vi "_readBoolSpecItem.vi"(7 "Error If Not Found":bool, 8 "error in (no error)":errorcluster, 9 "Default Value":bool, 10 "Name":string, 11 "Build Spec In":refnum<class "tBSONDocument.lvclass">) -> (0 "error out":errorcluster, 1 "Value":bool, 2 "Found":bool, 3 "Build Spec Out":refnum<class "tBSONDocument.lvclass">)   [LabVIEW 2013, in "LVAutomationListener.lvlib" / "LVAutomationListener.lvclass"]
uses:
  LVAutomationListener.lvclass
  BSON/tBSONDocument/tBSONDocument.lvclass
  _status.ctl
  BSON/tBSONDocument/getBooleanValue.vi
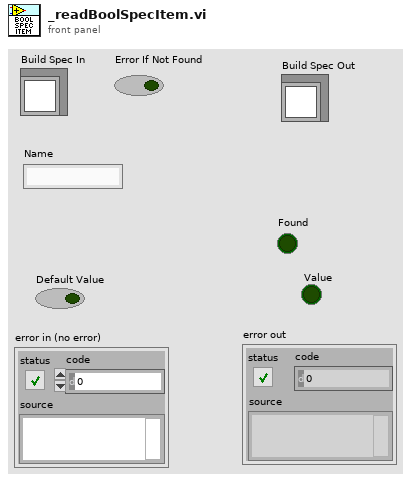
[diagram p1: front panel]
types:
  T1 = typedef "LVAutomationListener.lvlib/LVAutomationListener.lvclass/_status.ctl" = enum16{"Missing Argument", "Unknown Command", "Missing Build Spec Item", "Bad Type", "Compiler Aborted"}
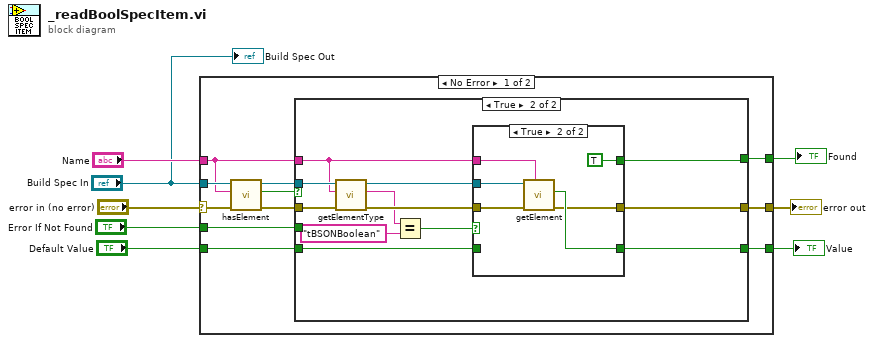
[diagram p0: block diagram]
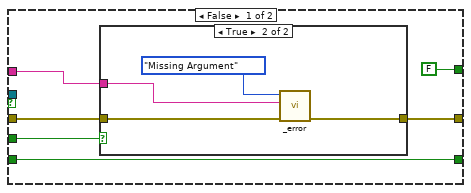
[diagram p2: hidden frame]
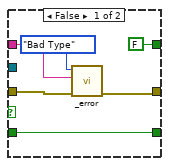
[diagram p4: hidden frame]
diagram:
  n1 = case shown="No Error" "error in (no error)" {
    selector: "error in (no error)" -> [w19 w56]
    tunnel: "Build Spec In" -> [w18 _]
    tunnel: "Name" -> [w13 _]
    tunnel: "Default Value" -> [w14 w55]
    tunnel: [w12 w55] -> w5
    tunnel: [w11 w56] -> w4
    tunnel: "Error If Not Found" -> [w10 _]
    tunnel: [w9 _] -> w1
    frame No Error {
      n2 = call "hasElement.vi"("error in (no error)"=w19, "Name"=w13, "tBSONDocument in"=w18) -> ("error out"=w16:errorcluster, "hasElement"=w17:bool, "tBSONDocument out"=w15:refnum<class "tBSONDocument.lvclass">)  [unwired: 6 in]
      n3 = case shown="True" w17 {
        tunnel: w16 -> [w23 w39]
        tunnel: w15 -> [_ w40]
        tunnel: w14 -> [w25 w34]
        tunnel: w13 -> [w22 w38]
        tunnel: [w25 w42] -> w12
        tunnel: [w21 w41] -> w11
        tunnel: w10 -> [w24 _]
        tunnel: [FALSE w33] -> w9
        frame False {
          n4 = case shown="True" w24 {
            tunnel: w23 -> [w26 w30]
            tunnel: w22 -> [_ w28]
            tunnel: [w26 w27] -> w21
            frame False {
            }
            frame True {
              n5 = call "_error.vi"("error in (no error)"=w30, "Additional message"=w28, "Status"=_status."Missing Argument") -> ("error out"=w27:errorcluster)  [unwired: 8 in]
            }
          }
        }
        frame True {
          n6 = call "getElementType.vi"("error in (no error)"=w39, "Name"=w38, "tBSONDocument in"=w40) -> ("error out"=w37:errorcluster, "TypeClass"=w31:string, "tBSONDocument out"=w36:refnum<class "tBSONDocument.lvclass">)  [unwired: 6 in]
          n7 = Equal?(x=w31, y="tBSONBoolean" ("x")) -> (x = y?=w35:bool)
          n8 = case shown="True" w35 {
            tunnel: [w44 w54] -> w42
            tunnel: [w45 w53] -> w41
            tunnel: w38 -> [w47 w52]
            tunnel: w37 -> [w48 w51]
            tunnel: w36 -> [_ w50]
            tunnel: w34 -> [w44 _]
            tunnel: [FALSE TRUE] -> w33
            frame False {
              n9 = call "_error.vi"("error in (no error)"=w48, "Additional message"=w47, "Status"=_status."Bad Type") -> ("error out"=w45:errorcluster)  [unwired: 8 in]
            }
            frame True {
              n10 = call-poly "getElement.vi"("Name"=w52, "error in (no error)"=w51, "tBSONDocument in"=w50) -> ("error out"=w53:errorcluster, "Value"=w54:bool)  [unwired: 6 in, 1 out]
            }
          }
        }
      }
    }
    frame Error {
    }
  }
  "error out" <- w4
  "Found" <- w1
  "Value" <- w5
  "Build Spec Out" <- "Build Spec In"
